vi "UpdateLimsTestStepAutomation.vi"(7 "step-id":u32, 8 "error in (no error)":errorcluster, 9 "instruction automation":string, 10 "link automation":string, 11 "ByteGSAPIBase in":refnum<class "ByteGSAPIBase.lvclass">) -> (0 "error out":errorcluster, 2 "step result":T1, 3 "ByteGSAPIBase out":refnum<class "ByteGSAPIBase.lvclass">)   [LabVIEW 2019, in "ByteGSWebAPI.lvlib" / "ByteGSAPIBase.lvclass"]
doc: "Update of automation link and instruction automation data based on step-id"
uses:
  ByteGSAPIBase.lvclass
  TypeDef/UpdateLimsTestStepData.ctl
  ByteGSAPIBase.lvclass/ByteGSAPIBase.ctl
  <vilib>/Bytelabs/ByteREST/ByteRESTClass/ByteRESTBase/RESTBase.lvclass
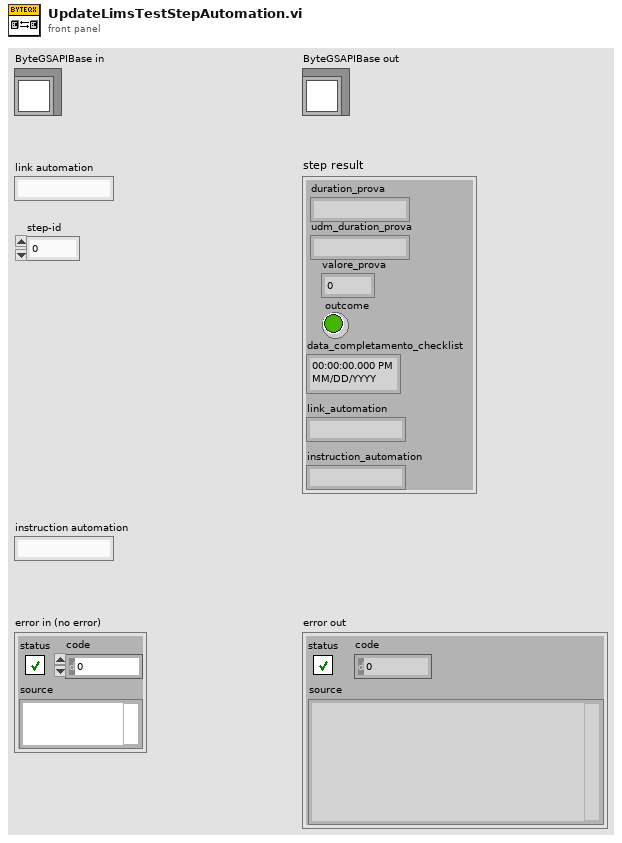
[diagram p1: front panel]
types:
  T1 = typedef "ByteGSWebAPI.lvlib/ByteGSAPIBase.lvclass/UpdateLimsTestStepData.ctl" = cluster{"outcome":bool, "data_completamento_checklist":timestamp, "udm_duration_prova":string, "valore_prova":dbl, "link_automation":string, "instruction_automation":string, "duration_prova":string}
  T2 = cluster{"link_automation":string, "instruction_automation":string, "udm_duration_prova":string, "outcome":string}
  T3 = cluster{"duration_prova":string, "udm_duration_prova":string, "data_completamento_checklist":string, "valore_prova":dbl, "outcome":string, "link_automation":string, "instruction_automation":string}
  T4 = typedef "ByteGSWebAPI.lvlib/ByteGSAPIBase.lvclass/Step.ctl" = cluster{"id":i32, "descrizione":string, "prova":string, "assets":T5[], "criterio_accettazione":string, "valore_criterio_accettazione_max":dbl, "valore_criterio_accettazione_min":dbl, "udm_criterio_accettazione":string, "duration_prova":string, "udm_duration_prova":string, "valore_prova":dbl, "ordine":i32, "user":i32, "link_automation":string, "instruction_automation":string, "data_completamento_checklist":timestamp, "outcome":bool}
  T5 = typedef "ByteGSWebAPI.lvlib/ByteGSAPIBase.lvclass/Asset.ctl" = cluster{"descrizione":string, "slug":string, "id":i32}
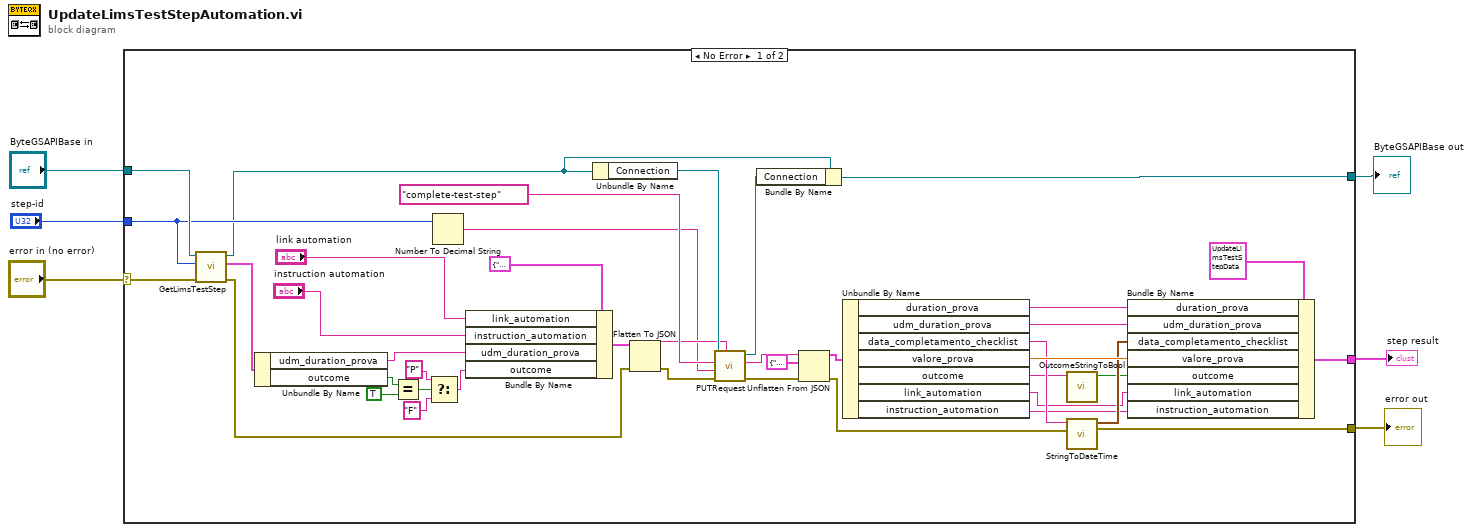
[diagram p0: block diagram]
diagram:
  n1 = case shown="No Error" "error in (no error)" {
    selector: "error in (no error)" -> [w20 w49]
    tunnel: [w32 w49] -> w5
    tunnel: [w46 w48] -> w3
    tunnel: "ByteGSAPIBase in" -> [w22 w48]
    tunnel: [w31 _] -> w2
    tunnel: "step-id" -> [w21 _]
    frame No Error {
      n2 = call-dynamic "GetLimsTestStep.vi"("error in (no error)"=w20, "step-id"=w21, "ByteGSAPIBase in"=w22) -> ("error out"=w19:errorcluster, "StepList"=w17:T4, "ByteGSAPIBase out"=w18:refnum<class "ByteGSAPIBase.lvclass">)  [unwired: 6 in]
      n3 = Unbundle By Name(w17) -> ("udm_duration_prova"=w16:string, "outcome"=w15:bool)
      n4 = Equal?(x=w15, y=TRUE) -> (x = y?=w13:bool)
      n5 = Select(t="P", s=w13, f="F") -> (s? t:f=w12:string)
      n6 = Number To Decimal String(number=w21) -> (decimal integer string=w25:string)  [unwired: 1 in]
      n7 = Bundle By Name(cluster=T2 {"link_automation"="", "instruction_automation"="", "udm_duration_prova"="", "outcome"=""}, "link_automation"="link automation", "instruction_automation"="instruction automation", "udm_duration_prova"=w16, "outcome"=w12) -> (w29:T2)
      n8 = Unbundle By Name(w18) -> ("Connection"=w47:refnum<class "RESTBase.lvclass">)
      n9 = Flatten To JSON(anything=w29, error in (no error)=w19) -> (JSON string=w43:string, 11:w42:errorcluster)  [unwired: 1 in]
      n10 = call-dynamic "PUTRequest.vi"("Body in"=w43, "error in (no error)"=w42, "Parameter"=w25, "Request"="complete-test-step", "ByteRESTBase in"=w47) -> ("error out"=w40:errorcluster, "Body"=w41:string, "ByteRESTBase out"=w45:refnum<class "RESTBase.lvclass">)  [unwired: 3 in, 1 out]
      n11 = Bundle By Name(cluster=w18, "Connection"=w45) -> (w46:refnum<class "ByteGSAPIBase.lvclass">)
      n12 = Unflatten From JSON(JSON string=w41, type and defaults=T3 {"duration_prova"="", "udm_duration_prova"="", "data_completamento_checklist"="", "valore_prova"=0.0, "outcome"="P", "link_automation"="", "instruction_automation"=""}, error in (no error)=w40) -> (value=w38:T3, error out=w28:errorcluster)  [unwired: 4 in]
      n13 = Unbundle By Name(w38) -> ("duration_prova"=w37:string, "udm_duration_prova"=w36:string, "data_completamento_checklist"=w34:string, "valore_prova"=w35:dbl, "outcome"=w8:string, "link_automation"=w27:string, "instruction_automation"=w26:string)
      n14 = call "OutcomeStringToBool.vi"("outcome string"=w8) -> ("outcome bool"=w7:bool)  [unwired: 10 in]
      n15 = call "StringToDateTime.vi"("error in (no error)"=w28, "datetime string"=w34) -> ("error out"=w32:errorcluster, "timestamp"=w33:timestamp)  [unwired: 8 in]
      n16 = Bundle By Name(cluster=T1 {"outcome"=FALSE, "data_completamento_checklist"=timestamp(0 s since 1904-01-01), "udm_duration_prova"="", "valore_prova"=0.0, "link_automation"="", "instruction_automation"="", "duration_prova"=""} ("Result Step"), "duration_prova"=w37, "udm_duration_prova"=w36, "data_completamento_checklist"=w33, "valore_prova"=w35, "outcome"=w7, "link_automation"=w27, "instruction_automation"=w26) -> (w31:T1)
    }
    frame Error {
    }
  }
  "error out" <- w5
  "ByteGSAPIBase out" <- w3
  "step result" <- w2
